vi "V_Gain.vi"(1 "Gain":T1) -> (0 "Gain (x)":dbl)   [LabVIEW 2016, in "KH7008.lvclass"]
uses:
  KH7008.lvclass
  typedefs/Gain-Enum.ctl
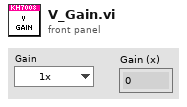
[diagram p1: front panel]
types:
  T1 = typedef "KH7008.lvclass/Gain-Enum.ctl" = enum16{"1x", "10x", "100x", "1000x"}
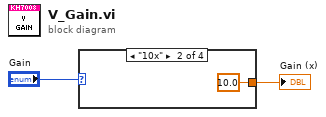
[diagram p0: block diagram]
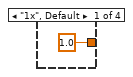
[diagram p2: hidden frame]
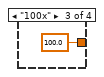
[diagram p3: hidden frame]
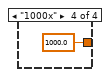
[diagram p4: hidden frame]
diagram:
  n1 = case shown="\"10x\"" "Gain" {
    tunnel: [1.0 ("y") 10.0 ("y") 100.0 ("y") 1000.0 ("y")] -> w2
    frame "1x", Default {
    }
    frame "10x" {
    }
    frame "100x" {
    }
    frame "1000x" {
    }
  }
  "Gain (x)" <- w2
